vi "Waveform chart & graph.vi"() -> ()   [LabVIEW 2022 SP3]
panel:
  out "Waveform Graph":dbl[](graph)
  in  "Stop Button":bool
  out "Celsius Chart":dbl(graph)
  out "Celsius":dbl
  in  "Fahrenheit":dbl
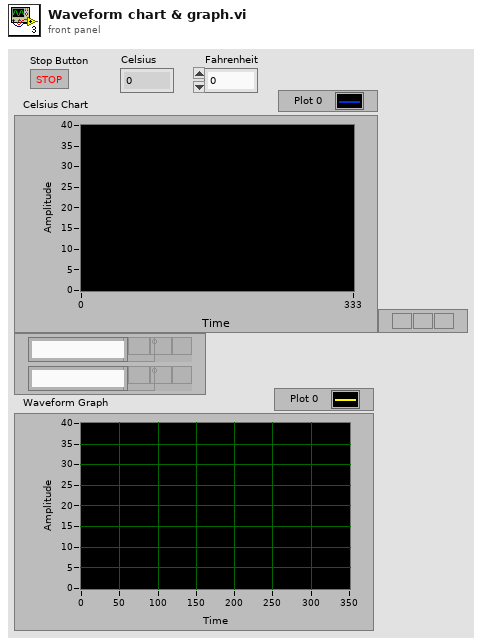
[diagram p1: front panel]
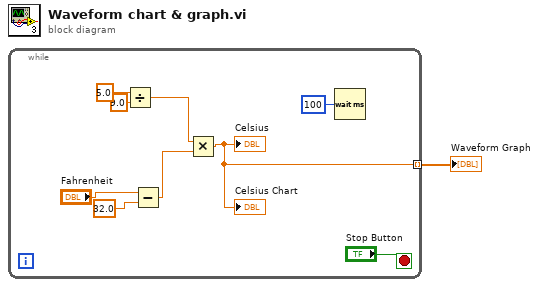
[diagram p0: block diagram]
diagram:
  n1 = while {
    tunnel: [w2] -> w1 mode=indexing
    stop <- "Stop Button" stop-if-true
    n2 = Divide(x=5.0, y=9.0) -> (x/y=w6:dbl)
    n3 = Subtract(x="Fahrenheit", y=32.0) -> (x-y=w5:dbl)
    n4 = Multiply(x=w6, y=w5) -> (x*y=w2:dbl)
    "Celsius" <- w2
    "Celsius Chart" <- w2
    n5 = Wait (ms)(milliseconds to wait=u32 100) -> ()  [unwired: 1 out]
  }
  "Waveform Graph" <- w1
